vi "Motor Speed Multiplier.vi"() -> ()   [LabVIEW 2017]
panel:
  in  "Turning Speed Multiplier":dbl=1.0
  in  "Straight Speed Multiplier":dbl=1.0
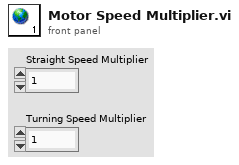
[diagram p1: front panel]
diagram:
